vi "基础8.vi"() -> ()   [LabVIEW 2014]
panel:
  out "ms":dbl
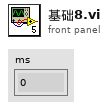
[diagram p1: front panel]
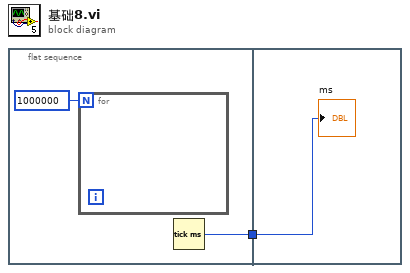
[diagram p0: block diagram]
diagram:
  n1 = flat-sequence {
    tunnel: [w3] -> w1
    tunnel: w1 -> [w4]
    frame #0 {
      n2 = for {
        N: 1000000 -> [_]
      }
      n3 = Tick Count (ms)() -> (millisecond timer value=w3:u32)
    }
    frame #1 {
      "ms" <- w4
    }
  }
